vi "play-raster-scan-via-CS.vi"() -> ()   [LabVIEW 2017]
uses:
  <vilib>/addons/Control Design/_Model Construction/Model Typedefs.llb/CD State Space Model (MIMO).ctl
  <vilib>/addons/Control Design/_Model Construction/Model Typedefs.llb/CD General Elements.ctl
  fpga_VIs/fpga_subVIs_ssxy/fixed-point-ss/typeDefs/FXPControlParams-ss-xy.ctl
  controls/z-axis-params_v4_prescan.ctl
  controls/TF-params.ctl
  controls/scan_input_meta_data.ctl
  controls/scan-mode-CTL.ctl
  fpga_VIs/controls/supervisor-params.ctl
  fpga_VIs/controls/fpga-scan-status.ctl
  controls/boolean_info.ctl
  <vilib>/userdefined/High Color/nirio_resource_hc.ctl
  controls/rasterMetaData_asCS.ctl
  <vilib>/FPGAPlugInAG/cRIO-9082/niLvFpga_Open_cRIO-9082.vi
  <vilib>/rvi/interface/common/dynamic/niFpgaDynamicAddResources.vi
  <vilib>/FPGAPlugInAG/Dynamic/niLvFpga_Reset_Dynamic.vi
  <vilib>/rvi/interface/common/niFpgaWaitOnOcc.vi
  <vilib>/Utility/error.llb/Error Cluster From Error Code.vi
  <vilib>/rvi/errors/niLvFpgaAdjustHostInterfaceError.vi
  <vilib>/FPGAPlugInAG/Dynamic/niLvFpga_Run_Dynamic.vi
  fpga_interface_lib/acquire_FXP_16-5_FIFO_2.vi
  <vilib>/RVI Host/nirviSupport.llb/nirviErrorClusterFromErrorCode.vi
  <vilib>/FPGAPlugInAG/Dynamic/niLvFpga_Close_Dynamic.vi
  <vilib>/rvi/interface/nirviOpenFPGA/nirviOpenFPGA.xnode
  FPGA Bitfiles/afmimagingcontro_FPGATargetSPARTA_cs-scanningv5ssx.lvbitx
  <vilib>/rvi/interface/nirviMethod/nirviMethod.xnode
  <vilib>/rvi/interface/nirviReadWriteControl/nirviReadWriteControl.xnode
  <vilib>/rvi/interface/nirviCloseFPGA/nirviCloseFPGA.xnode
  <vilib>/FPGAPlugInAG/Dynamic/niLvFpga_ConfigureFifo_Dynamic.vi
  <vilib>/rvi/errors/niLvFpgaMergeErrorWithErrorCode.vi
  <vilib>/rvi/interface/Simulation/niFpgaSimulationCallBeginRW.vi
  NiFpgaLv.dll
  fpga_interface_lib/fpga_interface.lvlib
  <vilib>/addons/_JKI.lib/Serialization/JSON/JKI JSON Serialization.lvlib
  <vilib>/rvi/interface/nirviMethod/StockFPGA_InlinedMethodWaitForSingleIRQ.vi
  <vilib>/FPGAPlugInAG/Dynamic/niLvFpga_WaitOnIrq_Dynamic.vi
  <vilib>/FPGAPlugInAG/Dynamic/niLvFpga_AcknowledgeIrq_Dynamic.vi
  <vilib>/FPGAPlugInAG/Dynamic/niLvFpga_WriteFifo_Dynamic.vi
  <vilib>/addons/Control Design/_Model Construction/NI_LinSys_Model Typedefs.lvlib
panel:
  out "state-counts":u64[](array[numeric])
  out "main iter":i32
  out "state0-count":u64
  out "output cluster":T1={"xy_settled_samples_threshold"=15, "xy_error_threshold"=0.01, "zup_err_threshold"=0.10000228881835938, "prescan_samples"=5000, "TOL"=0.3, "collect all"=TRUE, "numEntities"=0} {"TOL" format="%#_13g"}
  in  "number_of_scans":i64
  out "scan-idx":i16
  out "current-state":u8
  out "outer-iter":i32
  out "STOP 2":bool
  out "error out":errorcluster
  out "base x_ref(triangle wave)":dbl[](graph)
  out "base y_ref (ramp)":dbl[](graph)
  in  "Alert-on-Finish":bool
  out "state times":dbl[](array[numeric])
  out "ControlMatrices":T2
  in  "Tab Control":T3(tab)
  in  "input-data-path 2":path=path "Z:/afm-cs/imaging/raster/5microns/parents/raster_scan_128pix_5mic_01Hz.json"
  in  "z_axis_params":T4={"z_u_max"=5.0, "setpoint-scan"=-0.3000030517578125, "Ki-scan"=0.01, "uz_safe"=0.0, "Kiz_down"=0.02, "setpoint-up"=-0.899993896484375, "TF-params"={"TF-order"=0, "Num"=[0.0, 0.0, 0.0, 0.0, 0.0, 0.0, 0.0, 0.0, 0.0], "Den"=[0.0, 0.0, 0.0, 0.0, 0.0, 0.0, 0.0, 0.0, 0.0]}, "do-Dz"=FALSE, "PID-while-xy-move"=FALSE} {"Kiz_down" format="%#_13g"; "Ki-scan" min=0 max=0.4 step=0.0025; "z_u_max" format="%#_13g"}
  in  "overwrite":bool
  in  "input-data-path":path=path "Z:/afm-cs/imaging/raster/5microns/parents/raster_scan_128pix_5mic_01Hz.json"
  out "output-data-path":path
  in  "note-blob":string
  in  "state-machine-params":T1={"xy_settled_samples_threshold"=15, "xy_error_threshold"=0.01, "zup_err_threshold"=0.10000228881835938, "prescan_samples"=250, "TOL"=0.3, "collect all"=TRUE, "numEntities"=0} {"TOL" format="%#_13g"}
  in  "trigger-0":bool
  in  "STOP":bool
  out "CS Time":dbl
  in  "control_data_path":path=path "Z:/afm-cs/step-exps/LinControls01.json"
  in  "umax-xy":dbl=3.0 format="%#_13g"
  out "Gdrift-inv-xdir":T6 {"Transport Delay" format="%.2f"; "D" format="%#.5g"; "C" format="%#.5g"; "B" format="%#.5g"; "A" format="%#.5g"; "properties"."Sampling Time" format="%#.6p"; "properties"."Output Delays" format="%.4f"; "properties"."Input Delays" format="%.4f"}
  out "ControlParamsLin-ss":T8={"umax"=3.0, "Ns_obs/cntrl"=0, "ref_f_VEC"=[0.0, 0.0], "du_max"=0.0, "Nbar"=0.0, "Nhyst"=0, "Nsat"=0, "Ndrift+1"=0, "Ki-y"=0.01}
  in  "Ki-y":sgl=0.01
  out "scan-status":T9
  out "error out 2":errorcluster
  out "Actual Depth":u32
  out "scan_meta":T11
  out "output-meta-data-path":path
  # "make this come from input csv!"
  # "For the y-axis only, shouldnt ever really\nneed to change"
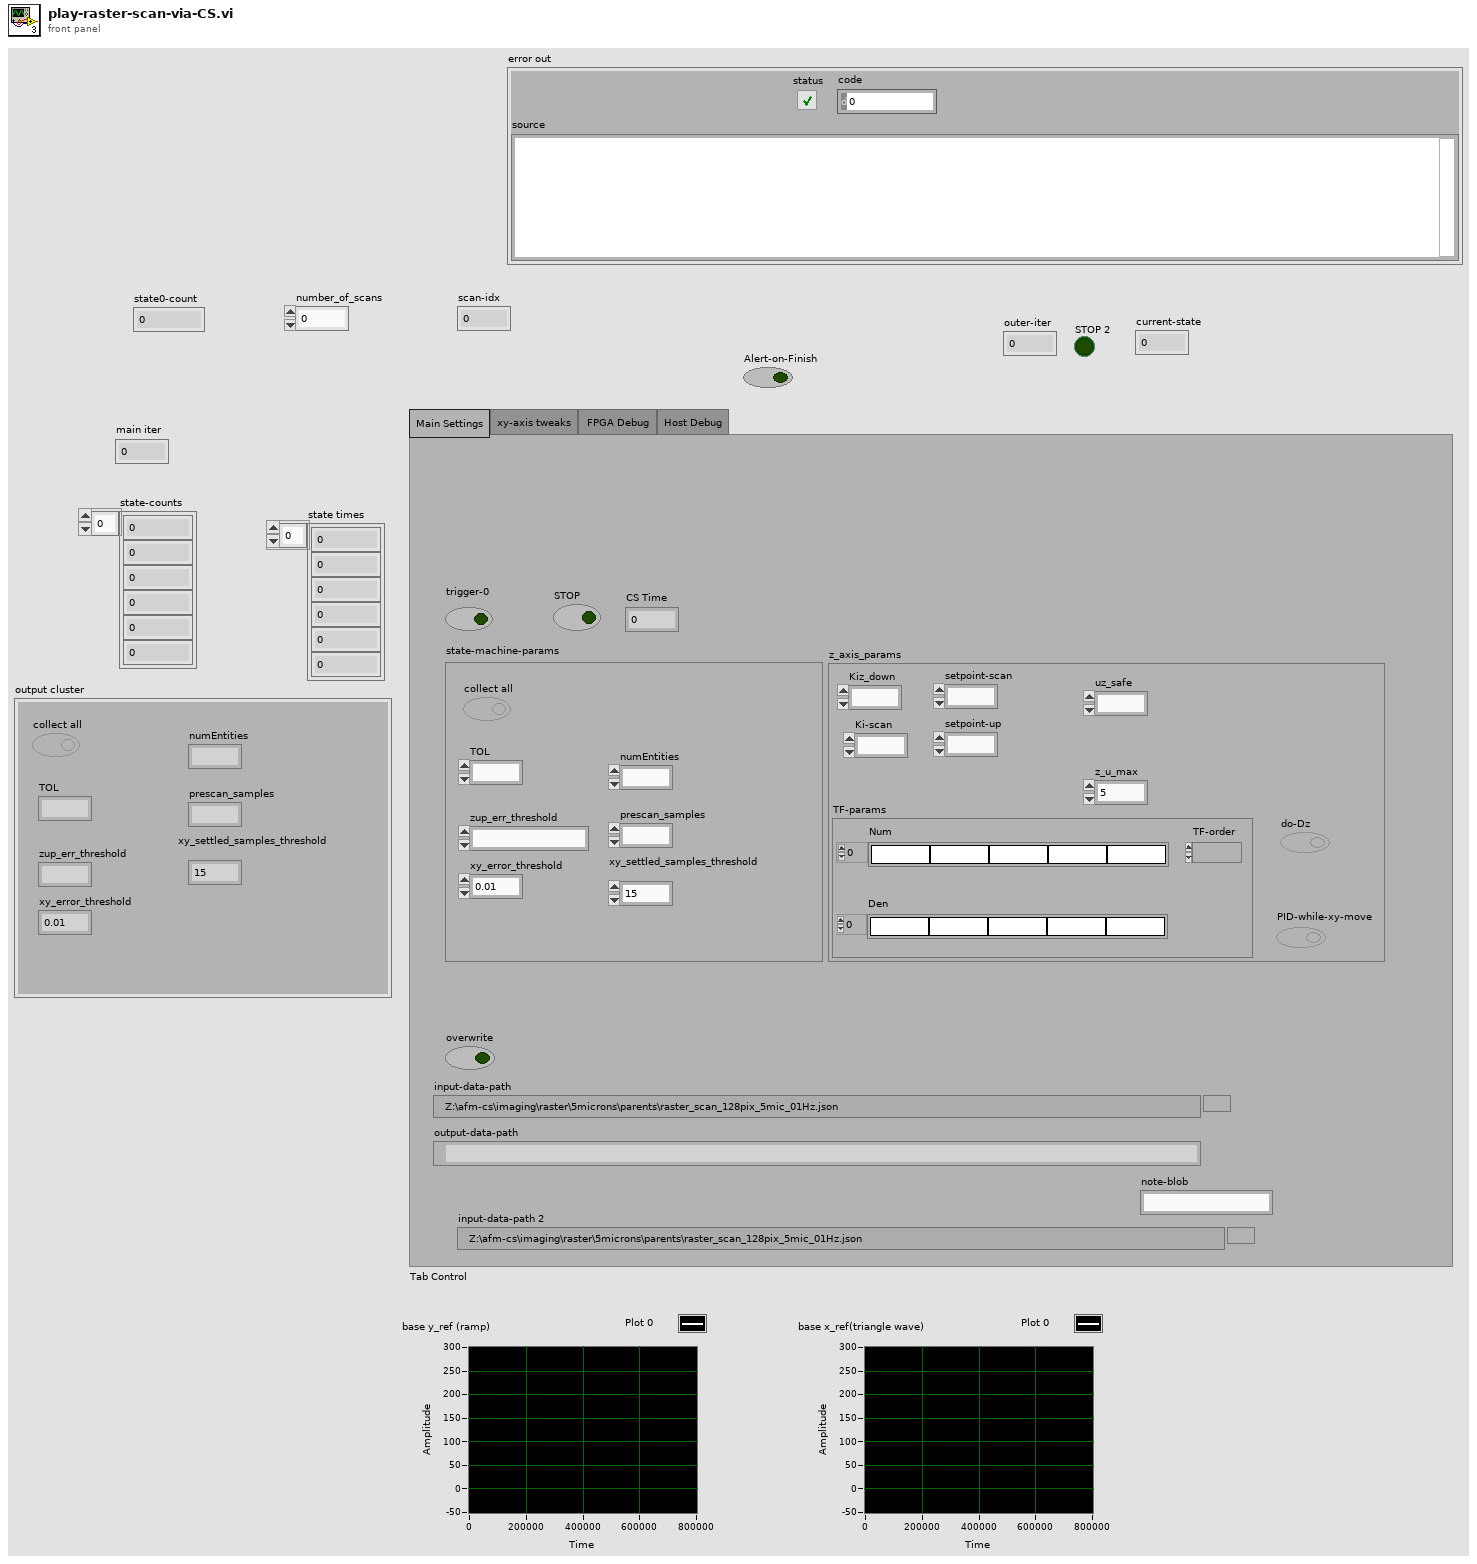
[diagram p1: front panel]
types:
  T1 = typedef "supervisor-params.ctl" = cluster{"xy_settled_samples_threshold":i16, "xy_error_threshold":sgl, "zup_err_threshold":fxp<+,24,5>, "prescan_samples":i16, "TOL":sgl, "collect all":bool, "numEntities":i16}
  T2 = cluster{"Az":fxp<+/-,32,4>[][], "Bz":dbl[][], "Lz":dbl[][], "Kz":dbl[][], "NxNu":dbl[][]}
  T3 = enum32{"Main Settings", "xy-axis tweaks", "FPGA Debug ", "Host Debug"}
  T4 = typedef "z-axis-params_v4_prescan.ctl" = cluster{"z_u_max":sgl, "setpoint-scan":fxp<+/-,32,16>, "Ki-scan":sgl, "uz_safe":fxp<+/-,16,5>, "Kiz_down":sgl, "setpoint-up":fxp<+/-,32,16>, "TF-params":T5, "do-Dz":bool, "PID-while-xy-move":bool}
  T5 = typedef "TF-params.ctl" = cluster{"TF-order":i16, "Num":sgl[], "Den":sgl[]}
  T6 = typedef "NI_LinSys_Model Typedefs.lvlib/CD State Space Model (MIMO).ctl" = cluster{"properties":T7, "A":dbl[][], "B":dbl[][], "C":dbl[][], "D":dbl[][], "StateNames":string[], "Transport Delay":dbl[][]}
  T7 = typedef "NI_LinSys_Model Typedefs.lvlib/CD General Elements.ctl" = cluster{"Model name":string, "Input names":string[], "Output names":string[], "Input Delays":dbl[], "Output Delays":dbl[], "Sampling Time":dbl, "Notes":string}
  T8 = typedef "FXPControlParams-ss-xy.ctl" = cluster{"umax":fxp<+/-,18,5>, "Ns_obs/cntrl":u8, "ref_f_VEC":fxp<+/-,32,5>[], "du_max":fxp<+/-,18,5>, "Nbar":fxp<+/-,32,5>, "Nhyst":u8, "Nsat":u8, "Ndrift+1":u8, "Ki-y":sgl}
  T9 = typedef "fpga-scan-status.ctl" = cluster{"boolean \nindicators":T10, "current-state":u8, "z-u(k)":sgl, "number-settled-samples-x":i16, "number-settled-samples-y":i16, "number-settled-samples-Z":i16, "scan-idx":i16, "state-counts":u64[]}
  T10 = typedef "boolean_info.ctl" = cluster{"unstable-z-traj":bool, "input fifo time-out":bool, "logging fifo timeout":bool, "scanning finished":bool, "unstable-x-traj":bool, "unstable-y-traj":bool, "ABORT":bool, "All Measurements Done":bool, "fpga_finished":bool}
  T11 = typedef "scan_input_meta_data.ctl" = cluster{"npix":i64, "raster_freq":dbl, "width":dbl, "points_per_line":i64, "points_per_period":i64, "total_num_points":i64, "scan_type":T12, "number_of_scans":i64, "actual_sub_samble_perc":dbl, "mu_length":dbl, "tip_velocity":dbl, "pix_idx":i32[]}
  T12 = typedef "scan-mode-CTL.ctl" = enum16{"raster", "CS"}
  T13 = typedef "nirio_resource_hc.ctl" = tag
  T14 = typedef "ObserverMatrices.ctl" = cluster{"Az":fxp<+/-,32,4>[][], "Bz":dbl[][], "Lz":dbl[][], "Kz":dbl[][], "NxNu":dbl[][]}
  T15 = typedef "rasterMetaData_asCS.ctl" = cluster{"Ki_xy":dbl, "number_of_lines":i32, "Ki-derate":sgl, "ze_sched_thresh":sgl, "scan_meta":T11, "z_axis_params":T4, "state_counts":dbl[], "state-machine-params":T1, "input-data-path":path, "output-data-path":path}
  T16 = enum16{"open", "replace", "create", "open or create", "replace or create", "replace or create with confirmation"}
  T17 = cluster{"boolean \nindicators":cluster{"unstable-z-traj":bool, "input fifo time-out":bool, "logging fifo timeout":bool, "scanning finished":bool, "unstable-x-traj":bool, "unstable-y-traj":bool, "ABORT":bool, "All Measurements Done":bool, "fpga_finished":bool}, "current-state":u8, "z-u(k)":sgl, "number-settled-samples-x":i16, "number-settled-samples-y":i16, "number-settled-samples-Z":i16, "scan-idx":i16, "state-counts":u64[]}
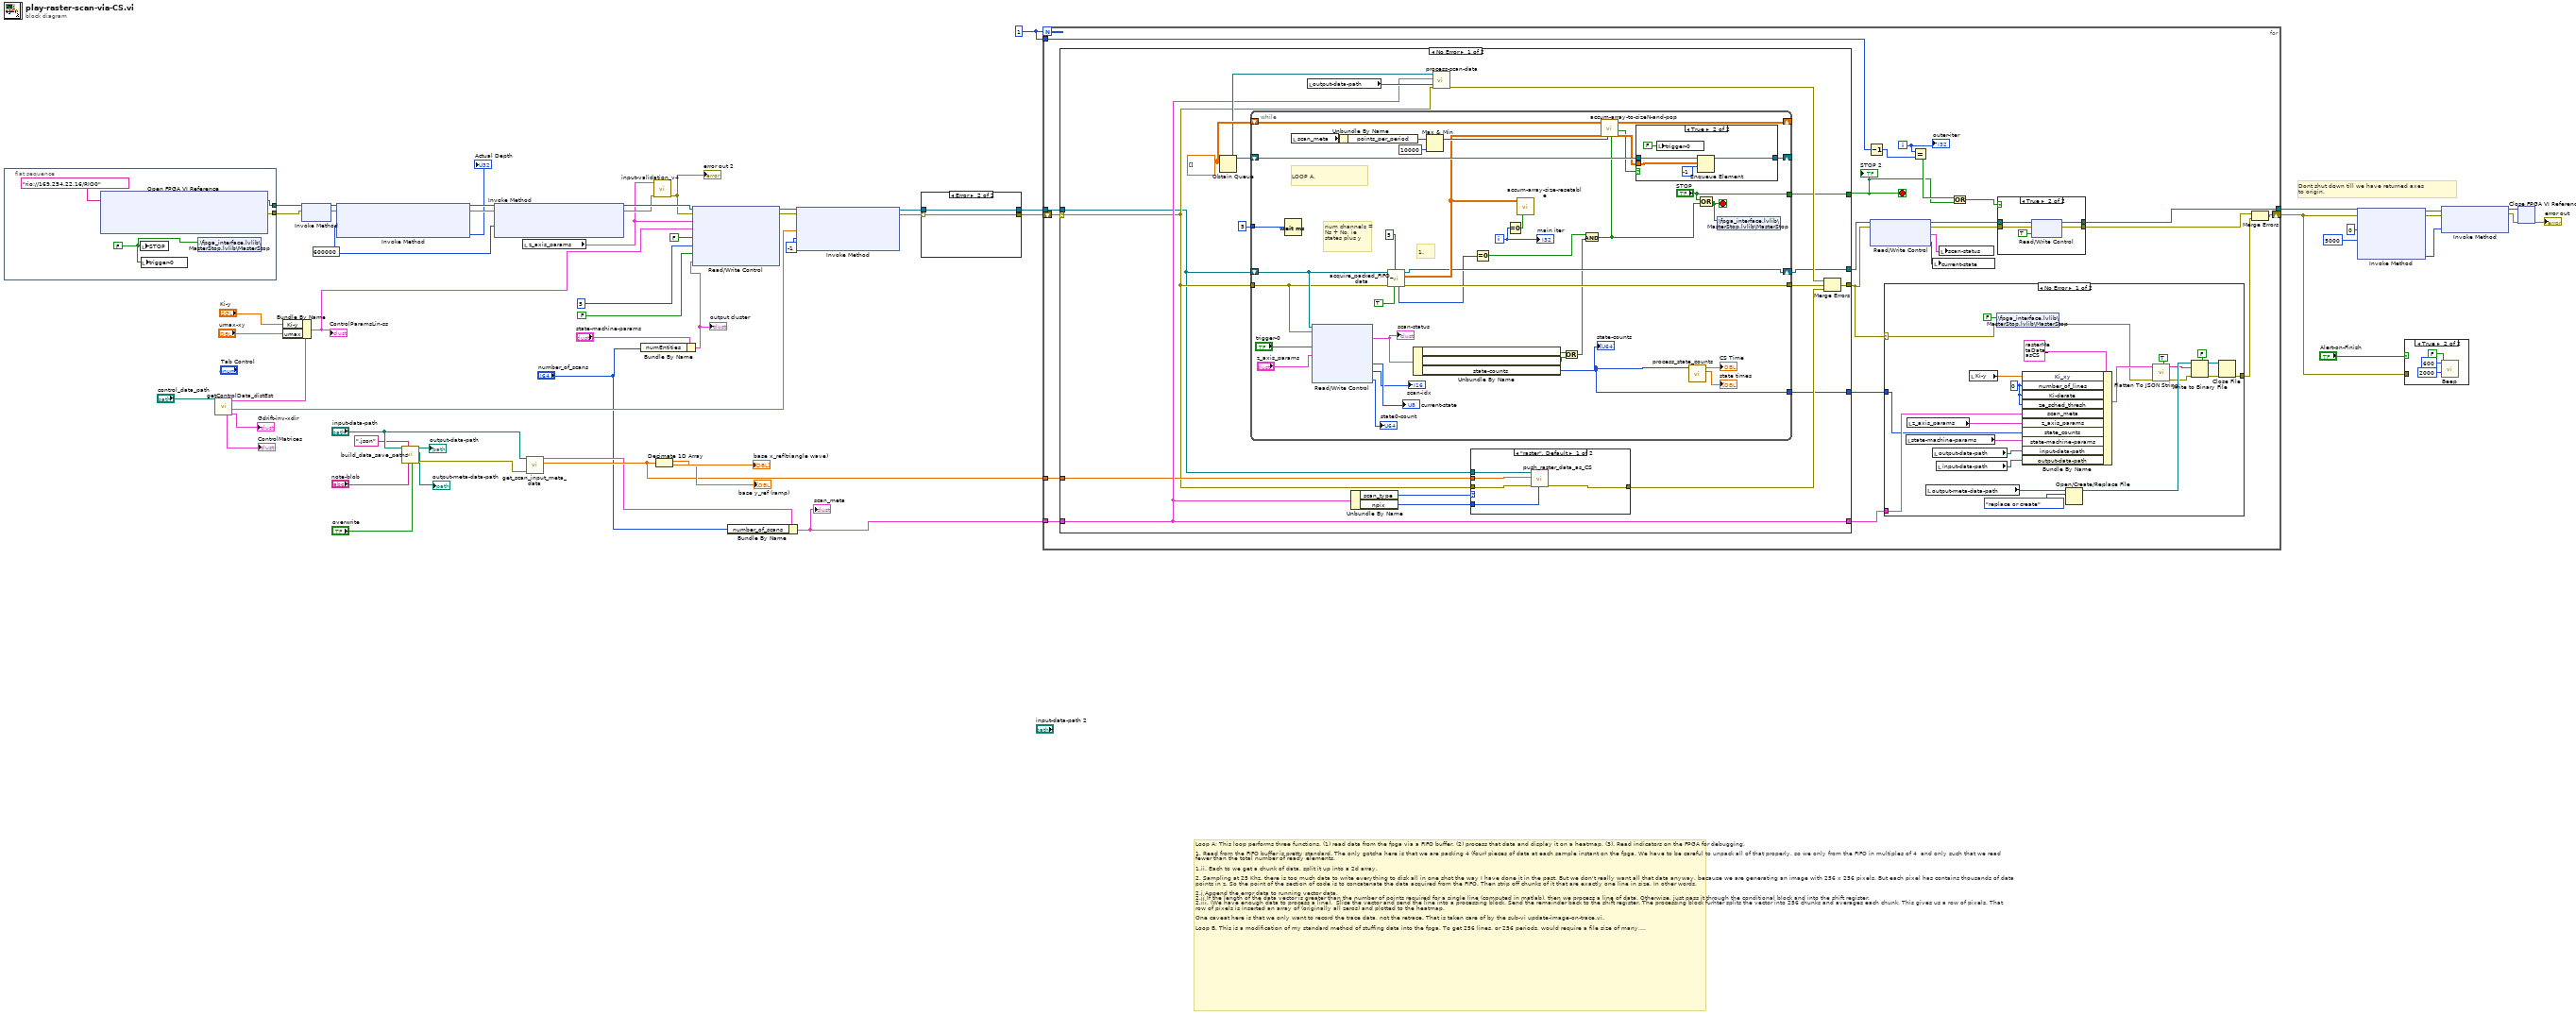
[diagram p0: block diagram]
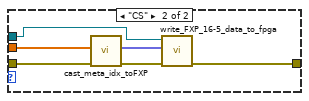
[diagram p5: hidden frame]
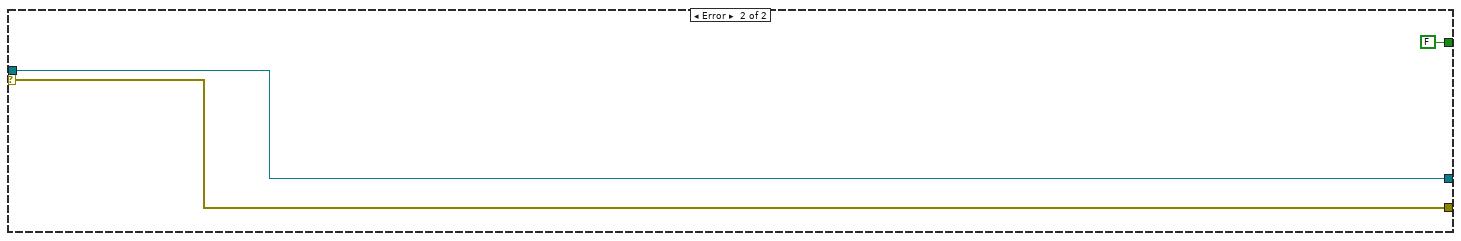
[diagram p7: hidden frame]
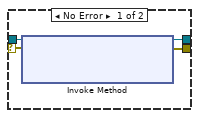
[diagram p8: hidden frame]
diagram:
  w4 = 1
  w57 = 600000
  # "Dont shut down till we have returned axes\nto origin."
  # "Loop A; This loop performs three functions. (1) read data from the fpga via a FIFO buffer. (2) process that data and display it on a heatmap. (3). Read indicators on the FPGA for debugging.\n\n1. Read from the FIFO buffer is pretty standard. The only gotcha here is that we are packing 4 (four) pieces of data at each sample instant on the fpga. We have to be careful to unpack all of that properly, so we only from the FIFO in multiples of 4  and only such that we read fewer than the total number of ready elements. \n\n1.ii. Each to we get a chunk of data, split it up into a 2d array. \n\n2. Sampling at 25 Khz, there is too much data to write everything to disk all in one shot the way I have done it in the past. But we don't really want all that data anyway, because we are generating an image with 256 x 256 pixels. But each pixel has contains thousands of data points in z. So the point of the section of code is to concatenate the data acquired from the FIFO. Then strip off chunks of it that are exactly one line in size. In other words,\n\n2.i Append the error data to running vector data.\n2.ii If the length of the data vector is greater than the number of points required for a single line (computed in matlab), then we process a line of data. Otherwise, just pass it through the conditional block and into the shift register. \n2.iii. (We have enough data to process a line).  Slice the vector and send the line into a processing block. Send the remainder back to the shift register. The processing block furhter splits the vector into 256 chunks and averages each chunk. This gives us a row of pixels. That row of pixels is inserted an array of (originally all zeros) and plotted to the heatmap.\n\nOne caveat here is that we only want to record the trace data, not the retrace. That is taken care of by the sub-vi update-image-on-trace.vi.\n\nLoop B. This is a modification of my standard method of stuffing data into the fpga. To get 256 lines, or 256 periods, would require a file size of many, many gigibtyes. SO the point here is to only use a single period of the triangle wave and corresponding ramp signal. Everytime we exauhst that data, re-cycle the same data and keep pumping it back in. The one tricky part here is that we have to be careful to shift the original ramp data up by the appropriate amount. We also have to take special care because of how the data is packed from matlab. [x(1), y(1), x(2), y(2)...].\n\nThe first iteration of the loop, we don't push any data in. All we do is get the number of empty elements.\n\nB.1 Each iteration, strip off ' empty elements ' elements from the array and send them to FIFO. \nB.2.i Is the remaining array empty?\nB.2.ii Grab the very last element. We need this"
  n1 = flat-sequence {
    tunnel: [w61] -> w56
    tunnel: [w60] -> w55
    frame #0 {
      w58 = FALSE
      n2 = xnode "Open FPGA VI Reference"("resource name"=T13 "rio://169.254.22.16/RIO0") -> ("FPGA VI Reference Out"=w61:refnum<k20>, "error out"=w60:errorcluster)  [unwired: 1 in]
      n3 = local write "STOP"(w58) -> ()
      n4 = local write "trigger-0"(w58) -> ()
      n5 = shared-variable ".\\fpga_interface.lvlib\\MasterStop.lvlib\\MasterStop"(w58) -> ()  [unwired: 1 in, 1 out]
    }
  }
  n6 = call "getControlData_distEst.vi"("system data path"="control_data_path") -> ("Gdrift"=→"Gdrift-inv-xdir":T6, "AllMatrix"=w33:dbl[], "ControlParams"=w44:T8, "ControlMatrices"=→"ControlMatrices":T14)  [unwired: 7 in]
  n7 = Bundle By Name(cluster=w44, "Ki-y"="Ki-y", "umax"="umax-xy") -> (w42:T8)
  "ControlParamsLin-ss" <- w42
  n8 = xnode "Invoke Method"("FPGA VI Reference In"=w56, "error in"=w55) -> ("FPGA VI Reference Out"=w52:refnum<k20>, "error out"=w51:errorcluster)
  n9 = xnode "Invoke Method"("FPGA VI Reference In"=w52, "error in"=w51, "Requested Depth"=w57) -> ("FPGA VI Reference Out"=w53:refnum<k20>, "error out"=w54:errorcluster, "Actual Depth"=→"Actual Depth":u32)
  n10 = call "build_data_save_paths.vi"("overwrite"="overwrite", "note-blob"="note-blob", "meta-file-ext"=".json" ("replace string (\"\")"), "input-file"="input-data-path") -> ("error IO"=w29:errorcluster, "output-meta-data-path"=→"output-meta-data-path":path, "output-data-path"=→"output-data-path":path)  [unwired: 4 in, 1 out]
  n11 = xnode "Invoke Method"("FPGA VI Reference In"=w53, "error in"=w54, "Requested Depth"=w57) -> ("FPGA VI Reference Out"=w46:refnum<k20>, "error out"=w41:errorcluster)  [unwired: 1 out]
  n12 = local read "z_axis_params"() -> (w25:T4)
  n13 = call "get_scan_input_meta_data.vi"("error in"=w29, "Path"="input-data-path") -> ("fpga_input"=w22:dbl[], "meta_data"=w3:T11)  [unwired: 7 in, 1 out]
  n14 = Bundle By Name(cluster="state-machine-params", "numEntities"="number_of_scans") -> (w23:T1)
  "output cluster" <- w23
  n15 = call "input-validation_v4.vi"("error constant"=w41, "z_axis_params"=w25) -> ("error out"=w40:errorcluster)  [unwired: 9 in]
  "error out 2" <- w40
  n16 = Decimate 1D Array(w22) -> (→"base x_ref(triangle wave)":dbl[], →"base y_ref (ramp)":dbl[])
  n17 = xnode "Read/Write Control"("FPGA VI Reference In"=w46, "error in"=w40, "z_axis_params"=w25, "ControlParams-ss-xy"=w42, "trigger-0"=FALSE, "num-log-channels"=u32 5 ("y"), "ABORT"=FALSE, "state-machine-params"=w23) -> ("FPGA VI Reference Out"=w36:refnum<k20>, "error out"=w35:errorcluster)
  n18 = Bundle By Name(cluster=w3, "number_of_scans"="number_of_scans") -> (w2:T11)
  "scan_meta" <- w2
  n19 = xnode "Invoke Method"("FPGA VI Reference In"=w36, "error in"=w35, "Data"=w33, "Timeout (ms)"=-1) -> ("FPGA VI Reference Out"=w18:refnum<k20>, "error out"=w19:errorcluster)  [unwired: 1 out]
  n20 = case shown="Error" w19 {
    selector: w19 -> [w65 w66]
    tunnel: w18 -> [w64 w67]
    tunnel: [w63 w66] -> w17
    tunnel: [w62 w67] -> w16
    frame No Error {
      n21 = xnode "Invoke Method"("FPGA VI Reference In"=w64, "error in"=w65) -> ("FPGA VI Reference Out"=w62:refnum<k20>, "error out"=w63:errorcluster)  [unwired: 1 in]
    }
    frame Error {
    }
  }
  n22 = for {
    N: w4 -> [_]
    tunnel: w2 -> [w88]
    tunnel: w22 -> [w87]
    shift-right: [w72] -> w7
    shift-left: w17 -> [w85]
    tunnel: w16 -> [w84]
    tunnel: [w73] -> w5
    tunnel: w4 -> [w79]
    i -> [w68]
    stop <- w77 stop-if-true
    n23 = case shown="No Error" w85 {
      selector: w85 -> [w124 w192]
      tunnel: [w135 w192] -> w80
      tunnel: [w121 w193] -> w83
      tunnel: w84 -> [w123 w193]
      tunnel: w88 -> [w129 _]
      tunnel: [w129 _] -> w89
      tunnel: w87 -> [w127 _]
      tunnel: [w125 _] -> w86
      tunnel: [w122 FALSE ("STOP")] -> w77
      frame No Error {
        w133 = dbl[][] []
        n24 = Obtain Queue(element data type=w133) -> (queue out=w131:refnum<queue>)  [unwired: 4 in, 2 out]
        n25 = while {
          tunnel: 5 -> [w185]
          tunnel: [w178] -> w136
          shift-right: [w182] -> _
          shift-left: w131 -> [w181]
          tunnel: w124 -> [w150]
          tunnel: [w163] -> w125
          shift-right: [w172] -> _
          shift-left: w133 -> [w171]
          tunnel: ["STOP"] -> w122
          shift-right: [w157] -> w121
          shift-left: w123 -> [w151]
          i -> [w160]
          stop <- w180 stop-if-true
          # "1."
          # "LOOP A."
          # "num channels = Ns + No, ie states plus y"
          n26 = Wait (ms)(milliseconds to wait=w185) -> ()  [unwired: 1 out]
          n27 = local read "scan_meta"() -> (w168:T11)
          n28 = xnode "Read/Write Control"("FPGA VI Reference In"=w151, "error in"=w150, "trigger-0"="trigger-0", "z_axis_params"="z_axis_params") -> ("scan-status"=w164:T17, "current-state"=→"current-state":u8, "scan-idx"=→"scan-idx":i16, "state0-count"=→"state0-count":u64)  [unwired: 2 out]
          "scan-status" <- w164
          n29 = Unbundle By Name(w168) -> ("points_per_period"=w167:i64)
          n30 = call-poly "acquire_packed_FIFO_data.vi"("Run once?"=TRUE, "numChannels"=u32 5 ("y"), "error in"=w150, "FPGA Interface(in)"=w151) -> ("error out"=w178:errorcluster, "2D Data Out"=w161:dbl[][], "FPGA VI Reference Out"=w157:refnum<k20>, "Elements Remaining"=w156:u32)  [unwired: 3 in, 1 out]
          n31 = Unbundle By Name(w164) -> ("boolean \nindicators.unstable-z-traj"=w184:bool, "boolean \nindicators.fpga_finished"=w183:bool, "state-counts"=w163:u64[])
          "state-counts" <- w163
          n32 = Max & Min(x=w167, y=i64 10000) -> (max(x,y)=w165:i64)  [unwired: 1 out]
          n33 = Equal To 0?(x=w156) -> (x = 0?=w155:bool)
          n34 = Equal To 0?(x=w160) -> (x = 0?=w159:bool)
          n35 = call "accum-array-size-resetable.vi"("reset"=w159, "array"=w161) -> ()  [unwired: 9 in, 1 out]
          n36 = Or(x=w184, y=w183) -> (x .or. y?=w154:bool)
          n37 = And(x=w155, y=w154) -> (x .and. y?=w149:bool)
          n38 = call "accum-array-to-sizeN-and-pop.vi"("flush"=w149, "Nsize"=w165, "new-data-in"=w161, "old-data-in"=w171) -> ("popped-data"=w170:dbl[][], "new-data-ready"=w169:bool, "old-data-out"=w172:dbl[][])  [unwired: 5 in]
          n39 = case shown="True" w169 {
            tunnel: w181 -> [w186 w191]
            tunnel: w170 -> [_ w189]
            tunnel: [w186 w188] -> w182
            frame False {
            }
            frame True {
              n40 = local write "trigger-0"(FALSE ("trigger-0")) -> ()
              n41 = Enqueue Element(queue=w191, element=w189, timeout in ms (-1)=-1) -> (queue out=w188:refnum<queue>)  [unwired: 1 in, 2 out]
            }
          }
          n42 = call "process_state_counts.vi"("state-counts"=w163) -> ("State_times"=→"state times":dbl[], "Cs_time"=→"CS Time":dbl)  [unwired: 9 in]
          n43 = Compound Arithmetic op=OR("STOP", w149) -> (w180:bool)
          n44 = shared-variable ".\\fpga_interface.lvlib\\MasterStop.lvlib\\MasterStop"(w180) -> ()  [unwired: 1 in, 1 out]
          "main iter" <- w160
        }
        n45 = local read "output-data-path"() -> (w130:path)
        n46 = Unbundle By Name(w129) -> ("scan_type"=w126:T12, "npix"=w132:i64)
        n47 = call "process-scan-data.vi"("error in"=w124, "output-data-path"=w130, "scan_meta"=w129, "queue in"=w131) -> ("error out"=w128:errorcluster)  [unwired: 7 in]
        n48 = case shown="\"raster\", Default" w126 {
          tunnel: [w142 w148] -> w134
          tunnel: w123 -> [w141 w143]
          tunnel: w132 -> [w140 _]
          tunnel: w124 -> [w139 w147]
          tunnel: w127 -> [w138 w144]
          frame "raster", Default {
            n49 = call "push_raster_data_as_CS.vi"("number-of-pixels"=w140, "error in"=w139, "fpga_input_vec"=w138, "FPGA Interface"=w141) -> ("error out"=w142:errorcluster)  [unwired: 6 in, 1 out]
          }
          frame "CS" {
            n50 = call "cast_meta_idx_toFXP.vi"("error in"=w147, "cs-traj-data-in"=w144) -> ("error out"=w146:errorcluster, "cs-traj-data-out"=w145:fxp<+/-,16,5>[])  [unwired: 8 in]
            n51 = call "write_FXP_16-5_data_to_fpga.vi"("error in"=w146, "all rows"=w145, "FPGA Interface"=w143) -> ("error out"=w148:errorcluster)  [unwired: 7 in, 1 out]
          }
        }
        n52 = Merge Errors(w128, w136, w134) -> (w135:errorcluster)
      }
      frame Error {
      }
    }
    "STOP 2" <- w77
    n53 = Decrement(x=w79) -> (x-1=w69:i32)
    n54 = xnode "Read/Write Control"("FPGA VI Reference In"=w83, "error in"=w80) -> ("FPGA VI Reference Out"=w75:refnum<k20>, "error out"=w74:errorcluster, "scan-status"=w81:T17, "current-state"=w82:u8)
    n55 = case shown="No Error" w80 {
      selector: w80 -> [w98 w120]
      tunnel: w89 -> [w111 _]
      tunnel: w86 -> [w101 _]
      tunnel: [w100 w120] -> w71
      frame No Error {
        w102 = 0 ("number_of_lines")
        n56 = local read "state-machine-params"() -> (w104:T1)
        n57 = local read "z_axis_params"() -> (w105:T4)
        n58 = local read "output-meta-data-path"() -> (w114:path)
        n59 = local read "output-data-path"() -> (w107:path)
        n60 = local read "input-data-path"() -> (w106:path)
        n61 = local read "Ki-y"() -> (w103:sgl)
        n62 = shared-variable ".\\fpga_interface.lvlib\\MasterStop.lvlib\\MasterStop"(FALSE ("MasterStop"), error in=w98) -> (error out=w97:errorcluster)
        n63 = Bundle By Name(cluster=T15 {"Ki_xy"=7.0, "number_of_lines"=0, "Ki-derate"=0.01, "ze_sched_thresh"=0.0, "scan_meta"={"npix"=0, "raster_freq"=0.0, "width"=0.0, "points_per_line"=0, "points_per_period"=0, "total_num_points"=0, "scan_type"=enum."raster", "number_of_scans"=0, "actual_sub_samble_perc"=0.0, "mu_length"=0.0, "tip_velocity"=0.0, "pix_idx"=[]}, "z_axis_params"={"z_u_max"=5.0, "setpoint-scan"=-0.3000030517578125, "Ki-scan"=0.02, "uz_safe"=0.0, "Kiz_down"=0.02, "setpoint-up"=-0.899993896484375, "TF-params"={"TF-order"=0, "Num"=[0.0, 0.0, 0.0, 0.0, 0.0, 0.0, 0.0, 0.0, 0.0], "Den"=[0.0, 0.0, 0.0, 0.0, 0.0, 0.0, 0.0, 0.0, 0.0]}, "do-Dz"=FALSE, "PID-while-xy-move"=FALSE}, "state_counts"=[], "state-machine-params"={"xy_settled_samples_threshold"=0, "xy_error_threshold"=0.01, "zup_err_threshold"=0.0, "prescan_samples"=-12144, "TOL"=256.0, "collect all"=TRUE, "numEntities"=256}, "input-data-path"=path "", "output-data-path"=path ""} ("raster_asCS__meta_out"), "Ki_xy"=w103, "number_of_lines"=w102, "Ki-derate"=w102, "ze_sched_thresh"=w102, "scan_meta"=w111, "z_axis_params"=w105, "state_counts"=w101, "state-machine-params"=w104, "input-data-path"=w107, "output-data-path"=w106) -> (w108:T15)
        n64 = Open/Create/Replace File(file path (use dialog)=w114, operation (0:open)=T16."replace or create") -> (refnum out=w116:refnum<file>)  [unwired: 4 in, 2 out]
        n65 = call <vilib>:"Flatten To JSON String.vi"("Numeric Extensions (F)"=TRUE, "error in (no error)"=w97, "Variant"=w108) -> ("error out"=w112:errorcluster, "JSON String"=w113:string)  [unwired: 7 in]
        n66 = Write to Binary File(file (use dialog)=w116, data=w113, error in=w112, 5:FALSE ("prepend array or string size? (T)")) -> (refnum out=w117:refnum<file>, error out=w118:errorcluster)  [unwired: 2 in, 1 out]
        n67 = Close File(refnum=w117, error in=w118) -> (error out=w100:errorcluster)  [unwired: 1 out]
      }
      frame Error {
      }
    }
    n68 = Equal?(x=w68, y=w69) -> (x = y?=w78:bool)
    n69 = local write "current-state"(w82) -> ()
    n70 = local write "scan-status"(w81) -> ()
    n71 = Or(x=w78, y=w77) -> (x .or. y?=w76:bool)
    n72 = case shown="True" w76 {
      tunnel: w75 -> [w91 w96]
      tunnel: w74 -> [w90 w95]
      tunnel: [w91 w94] -> w73
      tunnel: [w90 w93] -> w70
      frame False {
      }
      frame True {
        n73 = xnode "Read/Write Control"("FPGA VI Reference In"=w96, "error in"=w95, "ABORT"=TRUE) -> ("FPGA VI Reference Out"=w94:refnum<k20>, "error out"=w93:errorcluster)
      }
    }
    n74 = Merge Errors(w70, w71) -> (w72:errorcluster)
    "outer-iter" <- w68
  }
  n75 = xnode "Invoke Method"("FPGA VI Reference In"=w5, "error in"=w7, "IRQ Number(s)"=0, "Timeout (ms)"=5000) -> ("FPGA VI Reference Out"=w14:refnum<k20>, "error out"=w13:errorcluster, "IRQ(s) Asserted"=w15:i32)  [unwired: 1 out]
  n76 = case shown="True" "Alert-on-Finish" {
    tunnel: w7 -> [_ _]
    frame False {
    }
    frame True {
      n77 = call <vilib>:"Beep.vi"("use system alert? (T)"=FALSE, "duration (msec)"=u32 2000, "frequency (Hz)"=u32 600) -> ()  [unwired: 9 in]
    }
  }
  n78 = xnode "Invoke Method"("FPGA VI Reference In"=w14, "error in"=w13, "IRQ Number(s)"=w15) -> ("FPGA VI Reference Out"=w10:refnum<k20>, "error out"=w9:errorcluster)
  n79 = xnode "Close FPGA VI Reference"("FPGA VI Reference In"=w10, "error in"=w9) -> ("error out"=→"error out":errorcluster)
